vi "Timed Loop Synchronization.vi"() -> ()   [LabVIEW 2023]
doc: "Demonstrates the Synchronize to Scan Engine timing source to synchronize the Timed Loop to the period of the NI Scan Engine. This VI checks the Timed Loop for lateness and allows you to choose whether to set a major or minor fault upon detecting a late loop iteration."
uses:
  <vilib>/Platform/TimedLoop/XDataNode/timing_clust.ctl
  <vilib>/Platform/TimedLoop/XDataNode/nitl_modes.ctl
  <vilib>/Platform/TimedLoop/XDataNode/wakeup.ctl
  <vilib>/Platform/TimedLoop/XDataNode/loadnilvce.vi
  <vilib>/Platform/TimedLoop/XDataNode/XDataNode.xnode
  <vilib>/Platform/TimedLoop/XDataNode/XDNodeRunTimeDep.lvlib
panel:
  in  "Make Fault Major?":bool
  out "Loop Iterations":i32
  in  "Stop":bool
  in  "Wait Amount (ms)":u32(slide)=25 scale=0.0..250.0
  out "Loop Late?":bool
  in  "Scan Period (ms)":u32=100
  in  "Generate Fault on Late Loop Iterations?":bool
  # "Overview: This VI works similar to the While Loop Synchronization VI, except it uses the Synchronize to Scan Engine timing source to synchronize the Timed Loop to the period of the NI Scan Engine.  This VI checks the Timed Loop for lateness and allows you to choose whether to set a major or minor fault upon detecting a late loop iteration.  \nRequirements: LabVIEW Real-Time Module and NI-RIO driver\nInstructions:\n1. In Measurement & Automation Explorer, ensure that LabVIEW Real-Time and the NI Scan Engine are installed on your RT target.\n2. From the Project Explorer window, set the IP address of your RT target.\n3. Set the Scan Period (ms) front panel control of either the Timed Loop Synchronization.vi or While Loop Synchronization.vi to the desired loop rate. \n4. Run the VI in which you chose to set the Scan Period (mSec) control. \n5. Use the controls on the front panel to increase the wait amount in the While Loop. When you increase the wait amount beyond the scan period, the loop runs late and LabVIEW generates a fault.\n6. Run Fault Monitor.vi.\n7. Use the controls on the front panel to clear a specific fault code or to clear all faults.\n8. Click the Stop buttons on both VIs."
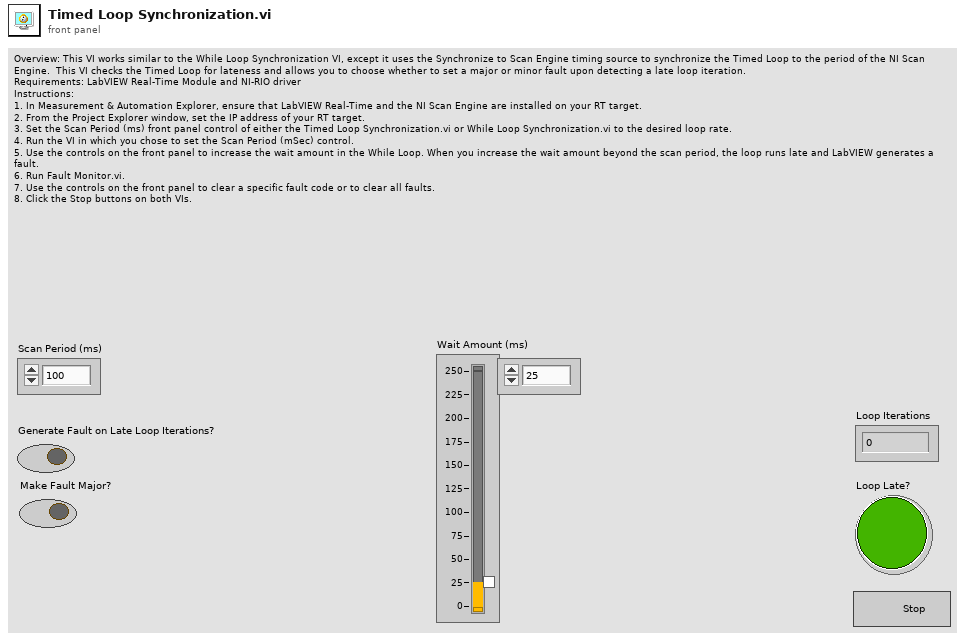
[diagram p1: front panel]
types:
  T1 = typedef "XDNodeRunTimeDep.lvlib/timing_clust.ctl" = cluster{"Expected End [f-1]":u64, "Actual End [f-1]":u64, "Finished Late? [f-1]":bool, "Expected End [i-1]":u64, "Actual End [i-1]":u64, "Finished Late? [i-1]":bool, "Expected Start [i]":u64, "Actual Start [i]":u64, "Expected Start [f]":u64, "Actual Start [f]":u64, "Source Name":string, "Structure Name":string, "Period":i64, "Deadline":i64, "Offset":i64, "Start":i64, "Priority":i32, "Timeout":i32, "Mode":T2, "Wakeup Reason":T3, "Error":errorcluster, "Source Type":string, "Secondary Source Type":string, "Global End Time":u64, "Global Start Time":u64, "Frame Duration":u64, "Iteration Duration":u64, "Assigned CPU":i32, "I/O Scan Engine Mode":u32}
  T2 = typedef "XDNodeRunTimeDep.lvlib/nitl_modes.ctl" = enum32{"No Change", "Process missed periods, maintain original phase", "Discard missed periods, maintain original phase", "Process missed periods, ignore original phase", "Discard missed periods, ignore original phase"}
  T3 = typedef "XDNodeRunTimeDep.lvlib/wakeup.ctl" = enum32{"Normal", "Aborted", "Asynchronous wakeup", "Timing source error", "Timed loop error", "Timeout"}
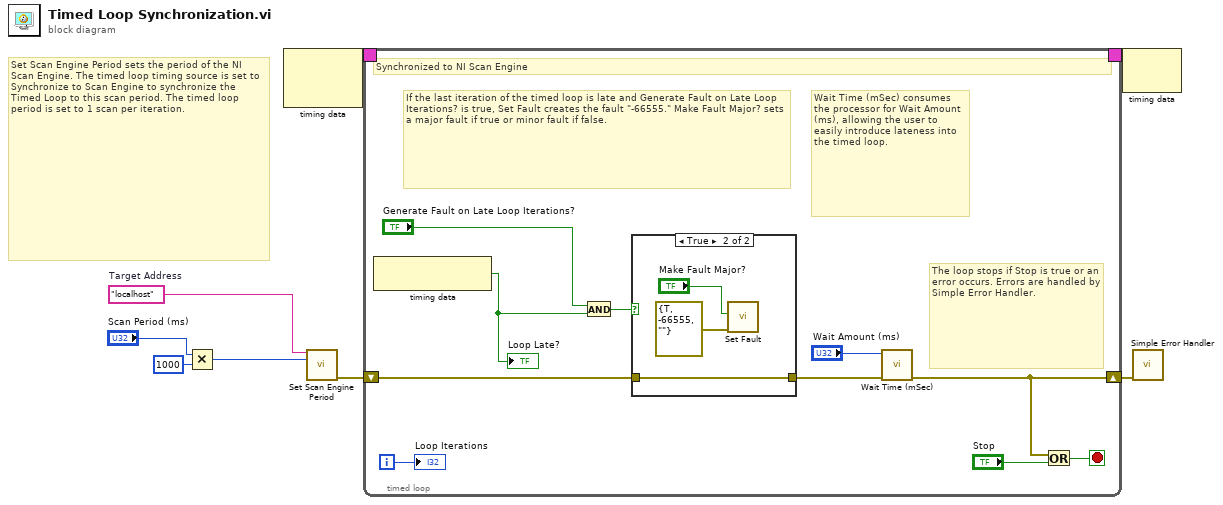
[diagram p0: block diagram]
diagram:
  w6 = "localhost"  # Target Address
  # "Set Scan Engine Period sets the period of the NI Scan Engine. The timed loop timing source is set to Synchronize to Scan Engine to synchronize the Timed Loop to this scan period. The timed loop period is set to 1 scan per iteration."
  n1 = Multiply(x="Scan Period (ms)", y=u32 1000) -> (x*y=w7:u32)
  n2 = node-c288() -> (w4:T1)  [unwired: 2 out]
  n3 = call <vilib>:"Set Scan Engine Period.vi"("target address (localhost)"=w6, "scan period (uSec)"=w7) -> ("error out"=w2:errorcluster)  [unwired: 1 in, 12 out]
  n4 = timed-loop {
    timing: w4 -> [_]
    timing-out: [_] -> w3
    shift-right: [w13] -> w1
    shift-left: w2 -> [w15]
    i -> [w18]
    stop <- w11 stop-if-true
    # "The loop stops if Stop is true or an error occurs. Errors are handled by Simple Error Handler."
    # "Wait Time (mSec) consumes the processor for Wait Amount (ms), allowing the user to easily introduce lateness into the timed loop."
    # "If the last iteration of the timed loop is late and Generate Fault on Late Loop Iterations? is true, Set Fault creates the fault \"-66555.\" Make Fault Major? sets a major fault if true or minor fault if false."
    # "Synchronized to NI Scan Engine"
    n5 = node-c288() -> (w9:bool)  [unwired: 1 out]
    "Loop Late?" <- w9
    n6 = And(x="Generate Fault on Late Loop Iterations?", y=w9) -> (x .and. y?=w17:bool)
    n7 = case shown="True" w17 {
      tunnel: w15 -> [w19 w20]
      tunnel: [w19 w20] -> w14
      frame False {
      }
      frame True {
        n8 = call <vilib>:"Set Fault.vi"("error in (user fault)"=errorcluster {"status"=TRUE, "code"=-66555, "source"=""}, "major fault (F)"="Make Fault Major?") -> ()  [unwired: 10 out]
      }
    }
    n9 = call "Wait Time (mSec).vi"("error in"=w14, "Spin Amount (mS)"="Wait Amount (ms)") -> ("error out"=w13:errorcluster)  [unwired: 9 in]
    n10 = Or(x=w13, y="Stop") -> (x .or. y?=w11:bool)
    "Loop Iterations" <- w18
  }
  n11 = node-c288(w3) -> ()  [unwired: 1 out]
  n12 = call <vilib>:"Simple Error Handler.vi"("error in (no error)"=w1) -> ()  [unwired: 1 in, 8 out]
